vi "Set_Maximum_DL_power.vi"(8 "error in (no error)":errorcluster, 9 "No of DL antennas Value":i32=-13 min=-64 max=-13, 10 "Cellular Technology":T1, 11 "Base Station":T2) -> (0 "error out":errorcluster, 3 "Output String":string)   [LabVIEW 2021]
uses:
  Controls/Base_Station_Emulator.ctl
  Controls/Cellular_Technology.ctl
  Controls/TCP_FGV.ctl
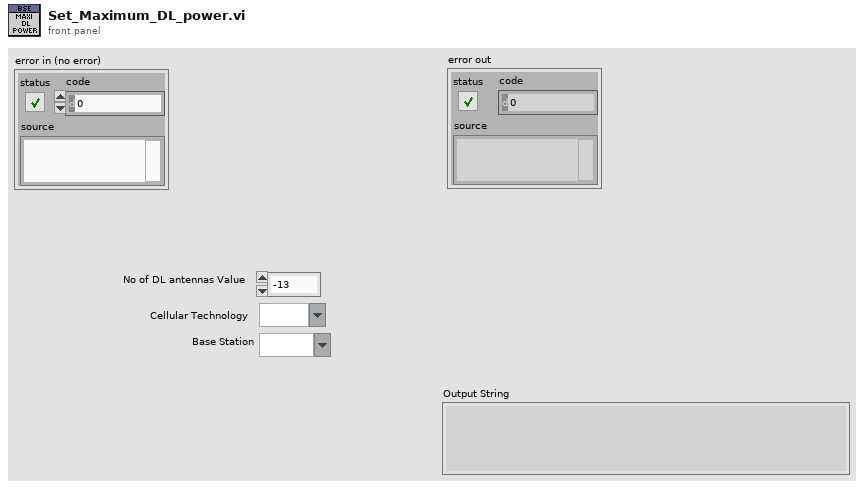
[diagram p1: front panel]
types:
  T1 = typedef "Cellular_Technology.ctl" = string
  T2 = typedef "Base_Station_Emulator.ctl" = string
  T3 = typedef "TCP_FGV.ctl" = enum16{"Open", "Read", "Write", "Close"}
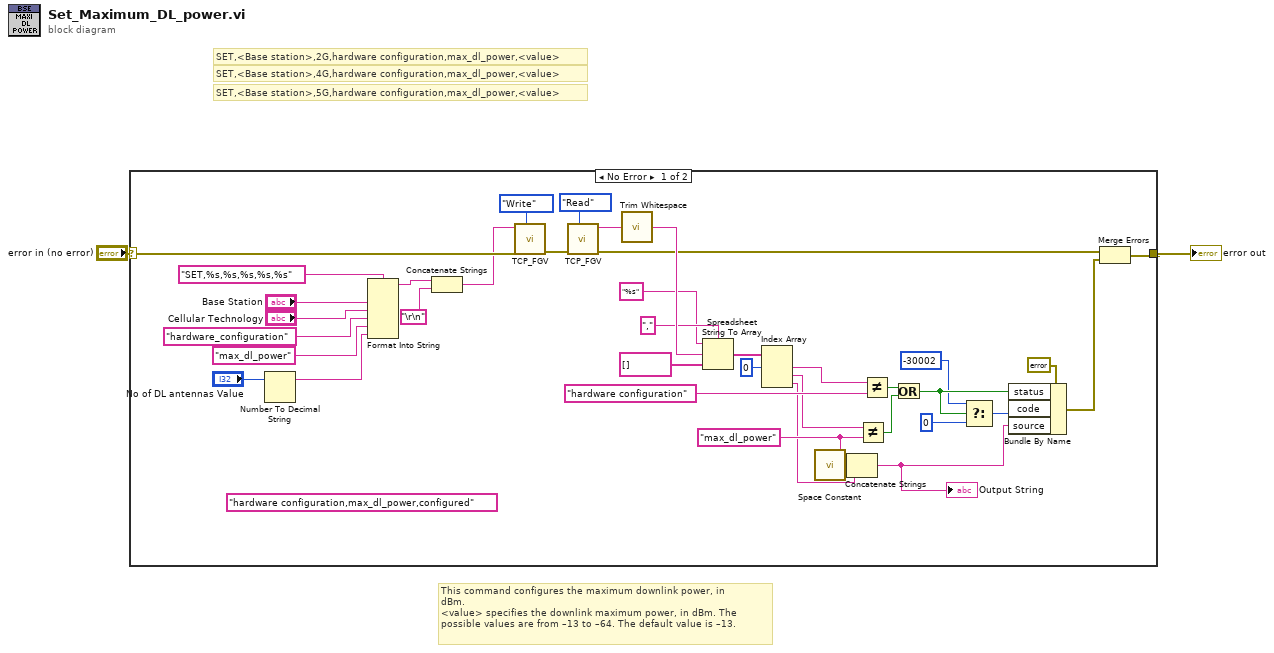
[diagram p0: block diagram]
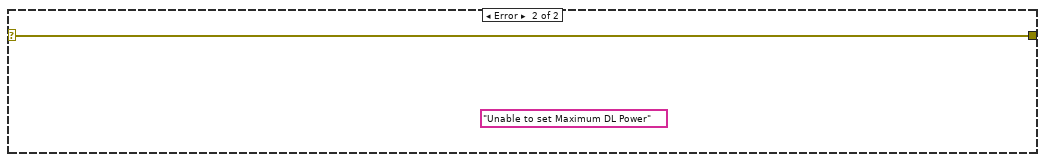
[diagram p2: hidden frame]
diagram:
  # "This command configures the maximum downlink power, in \ndBm. \n<value> specifies the downlink maximum power, in dBm. The \npossible values are from –13 to –64. The default value is –13."
  # "SET,<Base station>,5G,hardware configuration,max_dl_power,<value>"
  # "SET,<Base station>,4G,hardware configuration,max_dl_power,<value>"
  # "SET,<Base station>,2G,hardware configuration,max_dl_power,<value>"
  n1 = case shown="No Error" "error in (no error)" {
    selector: "error in (no error)" -> [w37 w41]
    tunnel: [w15 w41] -> w1
    frame No Error {
      (unwired) "hardware configuration,max_dl_power,configured" ("format string")
      w11 = "max_dl_power"
      n2 = Number To Decimal String(number="No of DL antennas Value") -> (decimal integer string=w6:string)  [unwired: 1 in]
      n3 = Format Into String(format string="SET,%s,%s,%s,%s,%s", "Base Station", "Cellular Technology", "hardware_configuration", "max_dl_power", w6) -> (resulting string=w4:string)  [unwired: 2 in, 1 out]
      n4 = Concatenate Strings(w4, "\r\n") -> (w3:string)
      n5 = call "TCP_FGV.vi"("Command"=w3, "error in (no error)"=w37, "Operation"=TCP_FGV."Write") -> ("error out"=w16:errorcluster)  [unwired: 6 in, 1 out]
      n6 = call "TCP_FGV.vi"("error in (no error)"=w16, "Operation"=TCP_FGV."Read") -> ("Data Out"=w13:string, "error out"=w18:errorcluster)  [unwired: 7 in]
      n7 = call <vilib>:"Trim Whitespace.vi"("string"=w13) -> ("trimmed string"=w29:string)  [unwired: 1 in]
      n8 = Spreadsheet String To Array(delimiter (Tab)=",", format string="%s", spreadsheet string=w29, array type (2D Dbl)=string[] []) -> (array=w33:string[])
      n9 = Index Array(array=w33, index #1=0 ("index")) -> (element #1=w32:string, element #2=w14:string, element #3=w10:string)  [unwired: 2 in]
      n10 = call <vilib>:"Space Constant.vi"() -> ("String"=w12:string)
      n11 = Concatenate Strings(w11, w12, w10) -> (w9:string)
      "Output String" <- w9
      n12 = Not Equal?(x=w14, y=w11) -> (x != y?=w30:bool)
      n13 = Not Equal?(x=w32, y="hardware configuration" ("format string")) -> (x != y?=w31:bool)
      n14 = Or(x=w31, y=w30) -> (x .or. y?=w28:bool)
      n15 = Select(t=-30002 ("code"), s=w28, f=0 ("code")) -> (s? t:f=w27:i32)
      n16 = Bundle By Name(cluster=errorcluster {"status"=FALSE, "code"=0, "source"=""} ("error constant"), "status"=w28, "code"=w27, "source"=w9) -> (w17:errorcluster)
      n17 = Merge Errors(w18, w17) -> (w15:errorcluster)
    }
    frame Error {
      (unwired) "Unable to set Maximum DL Power" ("source")
    }
  }
  "error out" <- w1
